vi "solar Create (SOLAR).vi"(8 "error in (no error)":errorcluster, 11 "solar in":refnum<class "solar.lvclass">) -> (0 "error out":errorcluster, 3 "solar out":refnum<class "solar.lvclass">)   [LabVIEW 2018, in "solar.lvclass"]
doc: "This launches the SOLAR user interface."
uses:
  solar.lvclass
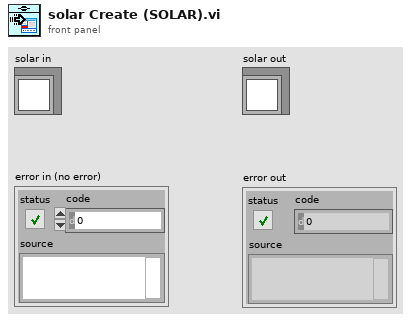
[diagram p1: front panel]
types:
  T1 = typedef "solar_ctl SOLAR Refnum.ctl" = refnum<k1>
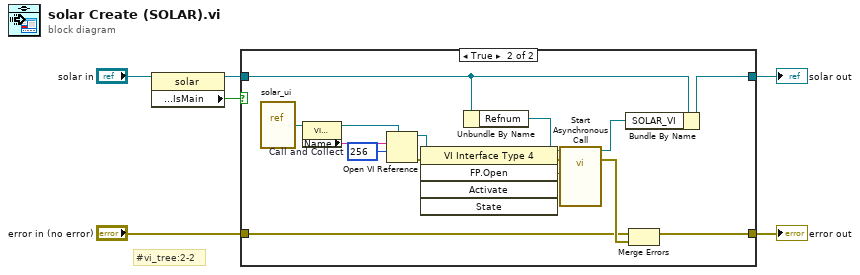
[diagram p0: block diagram]
diagram:
  # "#vi_tree:2-2"
  n1 = property class="solar"(reference="solar in") -> (reference out=w3:refnum<class "solar.lvclass">, "Accessors:Main.IsMain"=w2:bool)  [unwired: 1 in, 1 out]
  n2 = case shown="True" w2 {
    tunnel: "error in (no error)" -> [w7 w22]
    tunnel: [w7 w21] -> w4
    tunnel: w3 -> [w8 w12]
    tunnel: [w8 w10] -> w1
    frame False {
    }
    frame True {
      w17 = 256  # Call and Collect
      n3 = vi-ref "solar_ui.vi"() -> (w20:refnum<vi>)
      n4 = property class="VI (strict)"(reference=w20) -> (reference out=w18:refnum<vi>, "Name"=w19:string)  [unwired: 1 in, 1 out]
      n5 = Open VI Reference(type specifier VI Refnum (for type only)=w18, vi path=w19, options=w17) -> (vi reference=w14:refnum<vi>, error out=w16:errorcluster)  [unwired: 3 in]
      n6 = invoke class="VI Interface Type 4" method="FP.Open"(reference=w14, error in=w16) -> (reference out=w13:refnum<vi>, error out=w15:errorcluster)  [unwired: 3 in, 3 out]
      n7 = Unbundle By Name(w12) -> ("Refnum"=w11:T1)
      n8 = call-by-ref "Start Asynchronous Call"(reference=w13, error in=w15, "SOLAR Refnum"=w11) -> (reference out=w9:refnum<vi>, error out=w23:errorcluster)  [unwired: 11 in]
      n9 = Bundle By Name(cluster=w12, "SOLAR_VI"=w9) -> (w10:refnum<class "solar.lvclass">)
      n10 = Merge Errors(w22, w23) -> (w21:errorcluster)
    }
  }
  "error out" <- w4
  "solar out" <- w1
